vi "HeadersArrayToString.vi"(11 "additional headers (none)":T1[](array[typedef])) -> (3 "header string out":string)   [LabVIEW 2021, in "LV WebSockets.lvlib"]
doc: "Converts an array of headers to a string for inclusion in the HTTP header.\nWebSockets 1.6.0.22\nSam Sharp - MediaMongrels Ltd\nCopyright (c) 2016, MediaMongrels Ltd"
uses:
  LV WebSockets.lvlib
  Headers.ctl
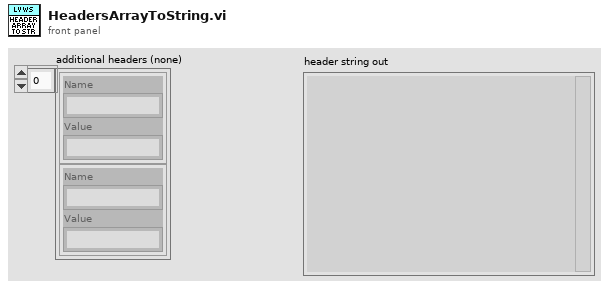
[diagram p1: front panel]
types:
  T1 = typedef "LV WebSockets.lvlib/Headers.ctl" = cluster{"Name":string, "Value":string}
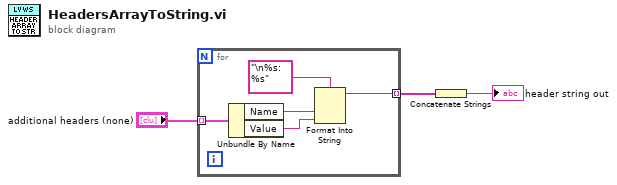
[diagram p0: block diagram]
diagram:
  n1 = for {
    tunnel: "additional headers (none)" -> [w8] mode=indexing
    tunnel: [w5] -> w2 mode=indexing
    n2 = Unbundle By Name(w8) -> ("Name"=w7:string, "Value"=w6:string)
    n3 = Format Into String(format string="\n%s: %s", w7, w6) -> (resulting string=w5:string)  [unwired: 2 in, 1 out]
  }
  n4 = Concatenate Strings(w2) -> (→"header string out":string)
